vi "Ctor.vi"(8 "error in (no error)":errorcluster) -> (0 "error out":errorcluster, 3 "Status out":refnum<class "Status.lvclass">)   [LabVIEW 2020, in "neg-pkg.lvlib" / "Status.lvclass"]
uses:
  Status.lvclass
  Status Message Data.ctl
  Status.lvclass/Status.ctl
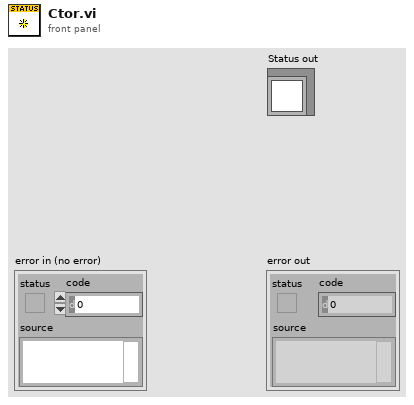
[diagram p1: front panel]
types:
  T1 = typedef "neg-pkg.lvlib/Status.lvclass/Status Message Data.ctl" = cluster{"Message":string}
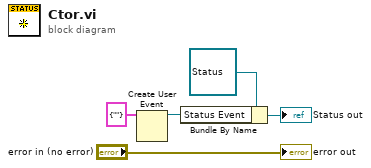
[diagram p0: block diagram]
diagram:
  n1 = Create User Event(user event datatype=T1 {"Message"=""} ("Status Message Data")) -> (user event=w1:refnum<user-event>)  [unwired: 1 in, 1 out]
  n2 = Bundle By Name(cluster=refnum<class "Status.lvclass"> refnum ("Status in"), "Status Event"=w1) -> (→"Status out":refnum<class "Status.lvclass">)
  "error out" <- "error in (no error)"
